vi "Scale Tags.vi"(11 "Scale Module Configs":T1[](array[typedef])) -> (1 "All Boolean Tags 2":string[](array[string]), 2 "Scale Tags Array":T5(array[cluster]), 3 "All  Numeric Tags 2":string[](array[string]))   [LabVIEW 2018]
uses:
  Scale Module Folder/Feed Module/Controls/Scale Module Config Cluster.ctl
  <vilib>/Utility/miscctls.llb/LVPoint32TypeDef.ctl
  Scale Module Folder/Feed Module/Controls/Scale Module Settings Cluster.ctl
  Mettler Toledo/Controls/Settings Cluster.ctl
  Mettler Toledo/Mettler Toledo.lvlib
  Scale Module Folder/Scale Module.lvlib
panel:
  # "Scale Settings"
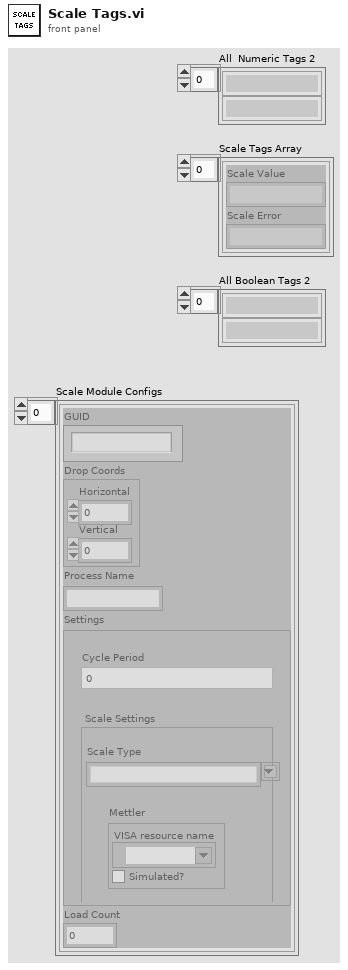
[diagram p1: front panel]
types:
  T1 = typedef "Scale Module.lvlib/Scale Module Config Cluster.ctl" = cluster{"GUID":string, "Drop Coords":T2, "Process Name":string, "Settings":T3, "Load Count":i32}
  T2 = typedef "LVPoint32TypeDef.ctl" = cluster{"Horizontal":i32, "Vertical":i32}
  T3 = typedef "Scale Module.lvlib/Scale Module Settings Cluster.ctl" = cluster{"Cycle Period":dbl, "Mettler":T4, "Scale Type":string}
  T4 = typedef "Mettler Toledo.lvlib/Settings Cluster.ctl" = cluster{"VISA resource name":refnum<visa-resource-name>, "Simulated?":bool}
  T5 = cluster{"Scale Value":string, "Scale Error":string}[]
  T6 = cluster{"Scale Value":string, "Scale Error":string}
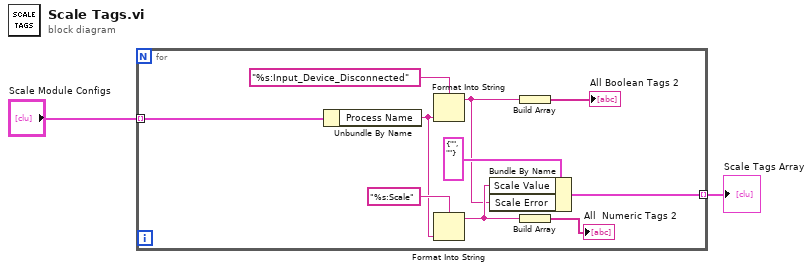
[diagram p0: block diagram]
diagram:
  n1 = for {
    tunnel: "Scale Module Configs" -> [w4] mode=indexing
    tunnel: [w5] -> w2 mode=indexing
    n2 = Unbundle By Name(w4) -> ("Process Name"=w3:string)
    n3 = Format Into String(format string="%s:Input_Device_Disconnected", w3) -> (resulting string=w6:string)  [unwired: 2 in, 1 out]
    n4 = Format Into String(format string="%s:Scale", w3) -> (resulting string=w8:string)  [unwired: 2 in, 1 out]
    n5 = Bundle By Name(cluster=T6 {"Scale Value"="", "Scale Error"=""} ("Scale Tags 2"), "Scale Value"=w8, "Scale Error"=w6) -> (w5:T6)
    n6 = Build Array(w6) -> (→"All Boolean Tags 2":string[])
    n7 = Build Array(w8) -> (→"All  Numeric Tags 2":string[])
  }
  "Scale Tags Array" <- w2
